vi "Generate Header Vectors.vi"(0 "RFFE Command in":refnum<class "RFFE Command.lvclass">, 11 "error in (no error)":errorcluster) -> (4 "RFFE Command out":refnum<class "RFFE Command.lvclass">, 6 "Header Vectors":string[](array[string]), 15 "error out":errorcluster)   [LabVIEW 2018, in "MIPI RFFE API.lvlib" / "RFFE Command.lvclass"]
uses:
  RFFE Command.lvclass
  RFFE Command.lvclass/RFFE Command.ctl
  Get Alias.vi
  Get Slave Address.vi
  Get Register Address.vi
  MIPI RFFE API.lvlib
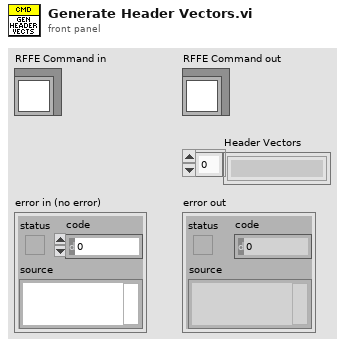
[diagram p1: front panel]
types:
  T1 = typedef "MIPI RFFE API.lvlib/Slave Address.ctl" = u8
  T2 = typedef "MIPI RFFE API.lvlib/Register Address.ctl" = u16
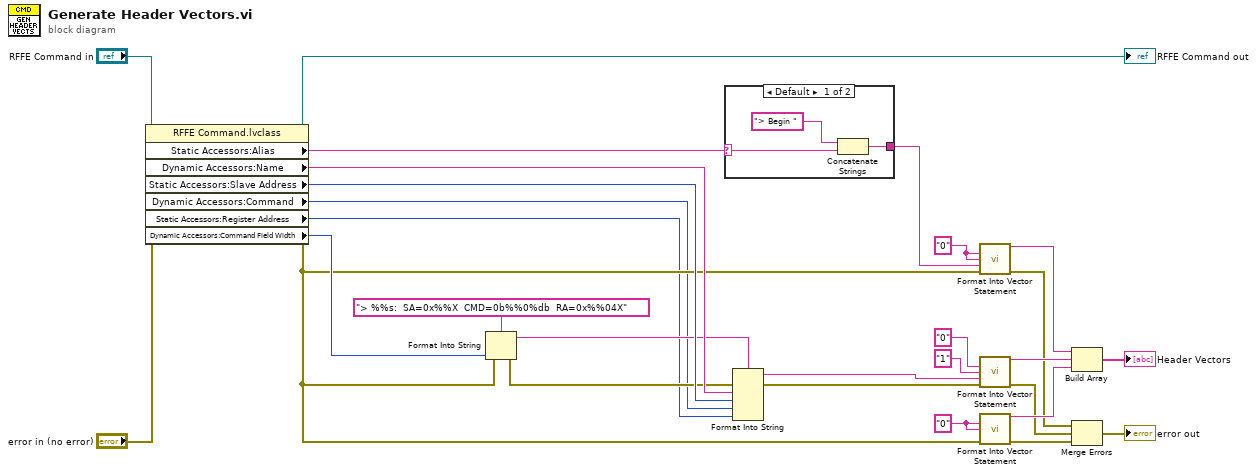
[diagram p0: block diagram]
diagram:
  w20 = "0" ("CLK")
  w26 = "0" ("CLK")
  n1 = property class="RFFE Command.lvclass"(reference="RFFE Command in", error in="error in (no error)") -> (reference out=→"RFFE Command out":refnum<class "RFFE Command.lvclass">, error out=w4:errorcluster, "Static Accessors:Alias"=w28:string, "Dynamic Accessors:Name"=w9:string, "Static Accessors:Slave Address"=w8:T1, "Dynamic Accessors:Command"=w2:u8, "Static Accessors:Register Address"=w1:T2, "Dynamic Accessors:Command Field Width"=w5:i32)
  n2 = Format Into String(format string="> %%s:  SA=0x%%X  CMD=0b%%0%db  RA=0x%%04X", error in=w4, w5) -> (resulting string=w6:string, error out=w3:errorcluster)  [unwired: 1 in]
  n3 = case shown="Default" w28 {
    selector: w28 -> [w31 _]
    tunnel: [w29 _] -> w18
    frame Default {
      n4 = Concatenate Strings("> Begin " ("CLK"), w31) -> (w29:string)
    }
    frame "" {
    }
  }
  n5 = Format Into String(format string=w6, error in=w3, w9, w8, w2, w1) -> (resulting string=w10:string, error out=w11:errorcluster)  [unwired: 1 in]
  n6 = call "Format Into Vector Statement.vi"("CLK (1)"=w20, "DATA (0)"=w20, "Comment"=w18, "error in (no error)"=w4) -> ("Vector Statement"=w17:string, "error out"=w19:errorcluster)  [unwired: 10 in]
  n7 = call "Format Into Vector Statement.vi"("CLK (1)"="0" ("CLK"), "DATA (0)"="1" ("CLK"), "Comment"=w10, "error in (no error)"=w11) -> ("Vector Statement"=w24:string, "error out"=w21:errorcluster)  [unwired: 10 in]
  n8 = call "Format Into Vector Statement.vi"("CLK (1)"=w26, "DATA (0)"=w26, "error in (no error)"=w4) -> ("Vector Statement"=w23:string, "error out"=w22:errorcluster)  [unwired: 11 in]
  n9 = Build Array(w17, w24, w23) -> (→"Header Vectors":string[])
  n10 = Merge Errors(w19, w21, w22) -> (→"error out":errorcluster)
